vi "oa_Buffer and Compute Timebase Plot Data.vi"(4 "interpolated pulse positions[s]":dbl[](array[numeric]) format="%.2f", 5 "reset? (F)":bool, 6 "trigger pulse direction":u16(ring)=1 items=["positive going", "negative going"], 7 "tach duty":i32=1, 8 "actual samples/rev":dbl format="%.2f", 9 "revolutions":dbl format="%.2f", 10 "start":dbl format="%.2f", 11 "order waveform":dbl[][](array[numeric]) format="%.2f") -> (2 "Y axis out":cluster{dbl[], dbl[]}[](array[cluster]) {"?" format="%.2f"; "?" format="%.2f"}, 3 "X axis out":cluster{dbl[], dbl[]}[](array[cluster]) {"?" format="%.2f"; "?" format="%.2f"})   [LabVIEW 2017]
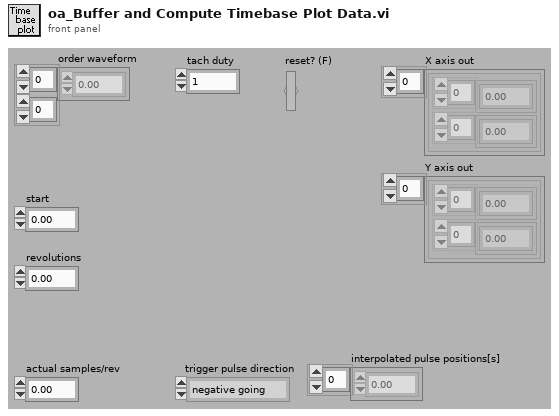
[diagram p1: front panel]
types:
  T1 = cluster{"selected order data":dbl[], "selected order data":dbl[]}
  T2 = cluster{"selected order data":dbl[], "selected order data":dbl[]}[]
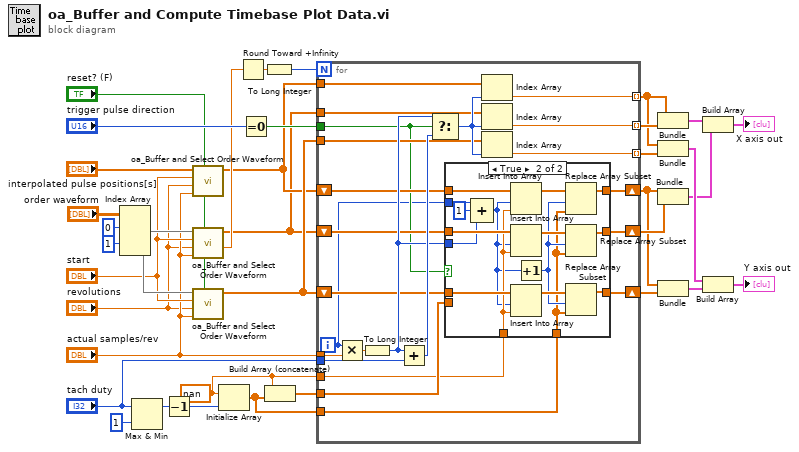
[diagram p0: block diagram]
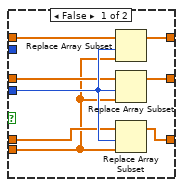
[diagram p2: hidden frame]
diagram:
  w17 = nan ("element")
  n1 = Index Array(array="order waveform", index (row) #1=0 ("index (row)"), index (row) #2=1 ("index (row)")) -> (element #1=w13:dbl[], element #2=w11:dbl[])  [unwired: 2 in]
  n2 = Max & Min(x="tach duty", y=1) -> (max(x,y)=w26:i32)  [unwired: 1 out]
  n3 = Decrement(x=w26) -> (x-1=w19:i32)
  n4 = call <vilib>:"oa_Buffer and Select Order Waveform.vi"("reset? (F)"="reset? (F)", "actual samples/rev"="actual samples/rev", "revolutions"="revolutions", "start"="start", "order data"="interpolated pulse positions[s]") -> ("selected order data"=w2:dbl[])  [unwired: 5 in, 1 out]
  n5 = call <vilib>:"oa_Buffer and Select Order Waveform.vi"("reset? (F)"="reset? (F)", "actual samples/rev"="actual samples/rev", "revolutions"="revolutions", "start"="start", "order data"=w13) -> ("rev out"=w5:dbl, "selected order data"=w1:dbl[])  [unwired: 5 in]
  n6 = call <vilib>:"oa_Buffer and Select Order Waveform.vi"("reset? (F)"="reset? (F)", "actual samples/rev"="actual samples/rev", "revolutions"="revolutions", "start"="start", "order data"=w11) -> ("selected order data"=w6:dbl[])  [unwired: 5 in, 1 out]
  n7 = Initialize Array(w17, w19) -> (w16:dbl[])
  n8 = Round Toward +Infinity(x=w5) -> (ceil(x): smallest int >= x=w3:dbl)
  n9 = Equal To 0?(x="trigger pulse direction") -> (x = 0?=w27:bool)
  n10 = To Long Integer(number=w3) -> (32bit integer=w36:i32)
  n11 = Build Array (concatenate)(w17, w16) -> (w18:dbl[])
  n12 = for {
    N: w36 -> [_]
    tunnel: "actual samples/rev" -> [w54]
    tunnel: [w57] -> w31 mode=indexing
    tunnel: [w56] -> w35 mode=indexing
    tunnel: [w55] -> w32 mode=indexing
    tunnel: w27 -> [w41]
    tunnel: "tach duty" -> [w53]
    shift-right: [w50] -> w23
    shift-left: w2 -> [w51]
    shift-right: [w48] -> w24
    shift-left: w1 -> [w45]
    shift-right: [w49] -> w22
    shift-left: w6 -> [w43]
    tunnel: w2 -> [w47]
    tunnel: w1 -> [w46]
    tunnel: w6 -> [w44]
    tunnel: w18 -> [w42]
    tunnel: w17 -> [w39]
    tunnel: w16 -> [w38]
    i -> [w40]
    n13 = Multiply(x=w40, y=w54) -> (x*y=w60:dbl)
    n14 = To Long Integer(number=w60) -> (32bit integer=w52:i32)
    n15 = Add(x=w52, y=w53) -> (x+y=w59:i32)
    n16 = Select(t=w52, s=w41, f=w59) -> (s? t:f=w58:i32)
    n17 = case shown="True" w41 {
      tunnel: w52 -> [w68 w70]
      tunnel: w51 -> [w67 w84]
      tunnel: [w66 w74] -> w50
      tunnel: [w65 w72] -> w49
      tunnel: [w64 w73] -> w48
      tunnel: w45 -> [w63 w83]
      tunnel: w43 -> [w62 w82]
      tunnel: w42 -> [w61 _]
      tunnel: w40 -> [_ w71]
      tunnel: w39 -> [_ w81]
      tunnel: w38 -> [_ w75]
      frame False {
        n18 = Replace Array Subset(array=w67, new element=w61, index=w68) -> (w66:dbl[])
        n19 = Replace Array Subset(array=w63, new element=w61, index=w68) -> (w64:dbl[])
        n20 = Replace Array Subset(array=w62, new element=w61, index=w68) -> (w65:dbl[])
      }
      frame True {
        n21 = Compound Arithmetic op=ADD(w71, 1 ("value"), w70) -> (w77:i32)
        n22 = Insert Into Array(array=w84, index=w77, new element=w81) -> (w80:dbl[])
        n23 = Insert Into Array(array=w83, index=w77, new element=w81) -> (w79:dbl[])
        n24 = Insert Into Array(array=w82, index=w77, new element=w81) -> (w78:dbl[])
        n25 = Increment(x=w77) -> (x+1=w76:i32)
        n26 = Replace Array Subset(array=w80, new element=w75, index=w76) -> (w74:dbl[])
        n27 = Replace Array Subset(array=w79, new element=w75, index=w76) -> (w73:dbl[])
        n28 = Replace Array Subset(array=w78, new element=w75, index=w76) -> (w72:dbl[])
      }
    }
    n29 = Index Array(array=w47, index=w58) -> (element=w57:dbl)
    n30 = Index Array(array=w46, index=w58) -> (element=w56:dbl)
    n31 = Index Array(array=w44, index=w58) -> (element=w55:dbl)
  }
  n32 = Bundle(w31, w35) -> (w34:cluster{dbl[], dbl[]})  [unwired: 1 in]
  n33 = Bundle(w31, w32) -> (w30:cluster{dbl[], dbl[]})  [unwired: 1 in]
  n34 = Bundle("selected order data"=w23, "selected order data"=w24) -> (w21:T1)  [unwired: 1 in]
  n35 = Bundle("selected order data"=w23, "selected order data"=w22) -> (w20:T1)  [unwired: 1 in]
  n36 = Build Array(w34, w21) -> (→"X axis out":T2)
  n37 = Build Array(w30, w20) -> (→"Y axis out":T2)
